vi "Initialise.vi"(8 "error in":errorcluster) -> (0 "error out":errorcluster, 1 "CAN Session":T1, 2 "interface object out":refnum<k20>, 3 "Log file":refnum<k34>)   [LabVIEW 2016]
uses:
  Motor controllers.vi
  Program Files (x86)/National Instruments/LabVIEW 2016/examples/robotics/EPOS2 CANOpen Driver/Low Level VIs/Typedefs/FPGA CAN Frame Cluster.ctl
  Program Files (x86)/National Instruments/LabVIEW 2016/examples/robotics/EPOS2 CANOpen Driver/Low Level VIs/Typedefs/Write Queue.ctl
  Program Files (x86)/National Instruments/LabVIEW 2016/examples/robotics/EPOS2 CANOpen Driver/Low Level VIs/Typedefs/kill process notifier array.ctl
  Program Files (x86)/National Instruments/LabVIEW 2016/examples/robotics/EPOS2 CANOpen Driver/Low Level VIs/Typedefs/CAN Communication References.ctl
  Program Files (x86)/National Instruments/LabVIEW 2016/examples/robotics/EPOS2 CANOpen Driver/Low Level VIs/Typedefs/CAN Session Pointer.ctl
  Program Files (x86)/National Instruments/LabVIEW 2016/examples/robotics/EPOS2 CANOpen Driver/Low Level VIs/Typedefs/CAN Refnum.ctl
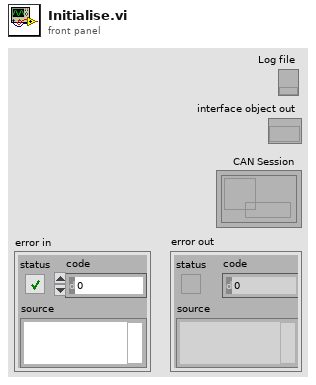
[diagram p1: front panel]
types:
  T1 = typedef "CAN Refnum.ctl" = refnum<k1>
  T2 = typedef "Log File Cluster.ctl" = cluster{"Log file":refnum<k34>, "semaphore":T3}
  T3 = typedef "Semaphore RefNum" = refnum<k1>
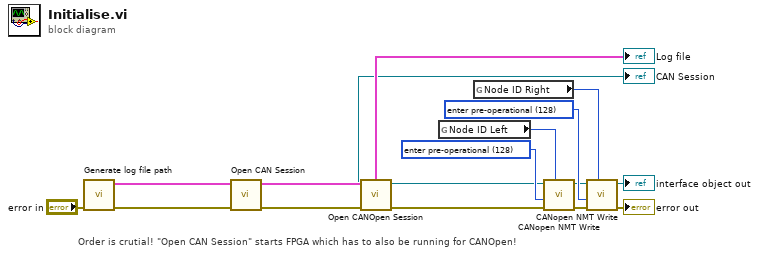
[diagram p0: block diagram]
diagram:
  w9 = u16 128 items=["start remote node"=1, "stop remote node"=2, "enter pre-operational"=128, "reset node"=129, "reset communication"=130] ("command")
  w10 = u16 128 items=["start remote node"=1, "stop remote node"=2, "enter pre-operational"=128, "reset node"=129, "reset communication"=130] ("command")
  # "Order is crutial! \"Open CAN Session\" starts FPGA which has to also be running for CANOpen!"
  n1 = call "Generate log file path.vi"("error in"="error in") -> ("error out"=w5:errorcluster, "Log File Cluster"=→"Log file":T2)  [unwired: 9 in]
  n2 = call "Open CAN Session.vi"("error in"=w5) -> ("error out"=w4:errorcluster, "CAN Session"=→"CAN Session":T1)  [unwired: 9 in]
  n3 = call "Open CANOpen Session.vi"("error in (no error)"=w4) -> ("error out"=w12:errorcluster, "interface object out"=w8:refnum<k20>)  [unwired: 9 in]
  n4 = global read "Motor controllers.vi" "Node ID Left"() -> (w14:u8)
  n5 = global read "Motor controllers.vi" "Node ID Right"() -> (w13:u8)
  n6 = call <vilib>:"CANopen NMT Write.vi"("node-ID (0)"=w14, "error in (no error)"=w12, "command"=w10, "interface object in"=w8) -> ("error out"=w11:errorcluster, "interface object out"=w7:refnum<k20>)  [unwired: 6 in]
  n7 = call <vilib>:"CANopen NMT Write.vi"("node-ID (0)"=w13, "error in (no error)"=w11, "command"=w9, "interface object in"=w7) -> ("error out"=→"error out":errorcluster, "interface object out"=→"interface object out":refnum<k20>)  [unwired: 6 in]
